vi "Unregister Status for Client.vi"(0 "CSM Name":string, 1 "TcpRouter-Client in":refnum<class "TcpRouter-Client.lvclass">, 5 "Source CSM Name":string="*", 11 "error in (no error)":errorcluster, 12 "Response Timeout(5000ms)":i32=5000) -> (4 "CSM Name(dup)":string, 15 "error out":errorcluster)   [LabVIEW 2020, in "CSM-TCP-Router.lvlib" / "TcpRouter-Client.lvclass"]
uses:
  TcpRouter-Client.lvclass
  _support/tcp-msg type.ctl
  bf4627cf-158a-4f4f-9b3b-34f06e1bff59.vi
  <userlib>/_NEVSTOP/Communicable State Machine(CSM)/AdvanceAPI/CSM - Revert Arguments-Safe String.vi
  <userlib>/_NEVSTOP/Communicable State Machine(CSM)/_Shared/Trim Single-line Text.vi
  <userlib>/_NEVSTOP/Communicable State Machine(CSM)/AdvanceAPI/CSM - Keywords.vi
  <userlib>/_NEVSTOP/Communicable State Machine(CSM)/_Polymophic/Build Unregister Message.vi
  TcpRouter-Client.lvclass/TcpRouter-Client.ctl
  CSM-TCP-Router.lvlib
  <userlib>/_NEVSTOP/Communicable State Machine(CSM)/Communicable State Machine.lvlib
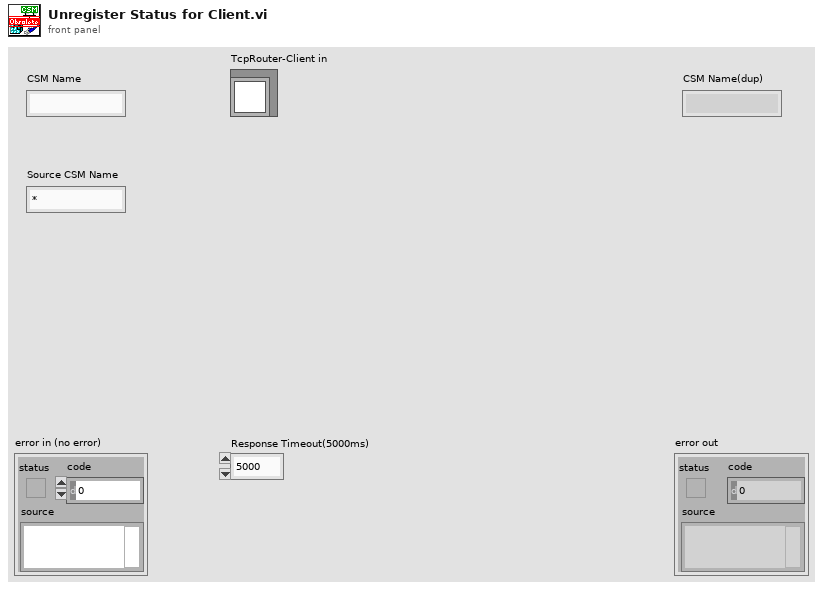
[diagram p1: front panel]
types:
  T1 = typedef "CSM-TCP-Router.lvlib/tcp-msg type.ctl" = enum8{"info", "error", "cmd", "cmd-resp", "resp", "async-resp", "status", "interrupt"}
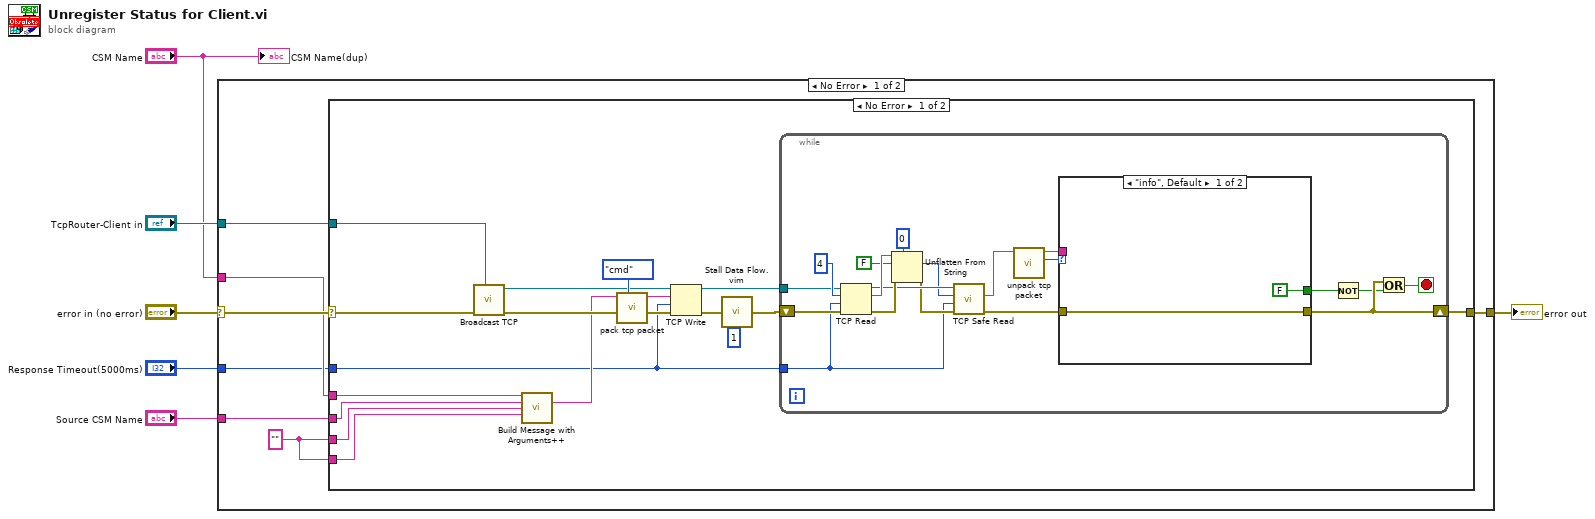
[diagram p0: block diagram]
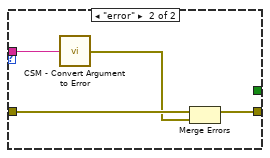
[diagram p2: hidden frame]
diagram:
  n1 = case shown="No Error" "error in (no error)" {
    selector: "error in (no error)" -> [w13 w57]
    tunnel: [w12 w57] -> w5
    tunnel: "TcpRouter-Client in" -> [w11 _]
    tunnel: "Response Timeout(5000ms)" -> [w8 _]
    tunnel: "CSM Name" -> [w10 _]
    tunnel: "Source CSM Name" -> [w9 _]
    frame No Error {
      w7 = "" ("Status")
      n2 = case shown="No Error" w13 {
        selector: w13 -> [w30 w56]
        tunnel: [w19 w56] -> w12
        tunnel: w11 -> [w29 _]
        tunnel: w8 -> [w18 _]
        tunnel: w10 -> [w17 _]
        tunnel: w9 -> [w16 _]
        tunnel: w7 -> [w15 _]
        tunnel: w7 -> [w14 _]
        frame No Error {
          n3 = call "Broadcast TCP.vi"("TcpRouter-Client in"=w29, "error in (no error)"=w30) -> ("error out"=w26:errorcluster, "connection ID"=w25:refnum<k5>)  [unwired: 8 in]
          n4 = call-poly <userlib>:"Build Message with Arguments++.vi"("Target CSM"=w17, "Source CSM (* as Default)"=w16, "Status"=w15, "API (* as Default)"=w14) -> ("CSM Message String"=w24:string)  [unwired: 11 in]
          n5 = call "pack tcp packet.vi"("tcp-message-type"=tcp-msg_type."cmd", "String"=w24) -> ("TCP Pack"=w28:string)  [unwired: 9 in]
          n6 = TCP Write(connection ID=w25, data in=w28, error in (no error)=w26, 9:w18) -> (connection ID out=w21:refnum<k5>, error out=w23:errorcluster)  [unwired: 1 out]
          n7 = call "Stall Data Flow.vim"("value in"=w23, "milliseconds to wait"=u32 1) -> ("value out"=w20:errorcluster)  [unwired: 1 out]
          n8 = while {
            tunnel: w21 -> [w40]
            shift-right: [w35] -> w19
            shift-left: w20 -> [w39]
            tunnel: w18 -> [w34]
            stop <- w33 stop-if-true
            n9 = TCP Read(connection ID=w40, bytes to read=4, error in (no error)=w39, 9:w34) -> (connection ID out=w47:refnum<k5>, data out=w48:string, error out=w49:errorcluster)  [unwired: 1 in]
            n10 = Unflatten From String(type=0, binary string=w48, data includes array or string size? (T)=FALSE, error in (no error)=w49) -> (value=w45:i32, error out=w44:errorcluster)  [unwired: 2 out]
            n11 = call "TCP Safe Read.vi"("error in (no error)"=w44, "timeout ms (25000)"=w34, "bytes to read"=w45, "TCP Network Connection in"=w47) -> ("error out"=w37:errorcluster, "String"=w46:string)  [unwired: 5 in, 1 out]
            n12 = call "unpack tcp packet.vi"("TCP Pack"=w46) -> ("tcp-message-type"=w38:T1, "String"=w36:string)  [unwired: 9 in]
            n13 = case shown="\"info\", Default" w38 {
              tunnel: w37 -> [w51 w55]
              tunnel: [w51 w53] -> w35
              tunnel: w36 -> [_ w54]
              tunnel: [FALSE _] -> w32
              frame "info", Default {
              }
              frame "error" {
                n14 = call <userlib>:"CSM - Convert Argument to Error.vi"("Argument"=w54) -> ("Error"=w52:errorcluster)  [unwired: 4 in]
                n15 = Merge Errors(w55, w52) -> (w53:errorcluster)
              }
            }
            n16 = Not(x=w32) -> (.not. x?=w31:bool)
            n17 = Or(x=w35, y=w31) -> (x .or. y?=w33:bool)
          }
        }
        frame Error {
        }
      }
    }
    frame Error {
    }
  }
  "error out" <- w5
  "CSM Name(dup)" <- "CSM Name"
